vi "parseSDfeatures.vi"(0 "binary[0] string":string, 1 "binary[1] string":string) -> (9 "RESISTANCE":string, 10 "WAHOO":string, 11 "BLE":string, 12 "DEMO":string, 13 "BUZZER":string, 14 "TV":string, 15 "AUDIO":string, 16 "USB":string, 17 "FAN":string, 18 "DMK":string, 19 "DISTANCE":string, 20 "CSAFE":string, 21 "SPEED":string, 22 "byte[1] array":string[](array[string]), 23 "GRADE":string, 24 "TABLET":string, 25 "byte[0] array":string[](array[string]), 26 "PULSE":string)   [LabVIEW 2018]
uses:
  Global_1259.vi
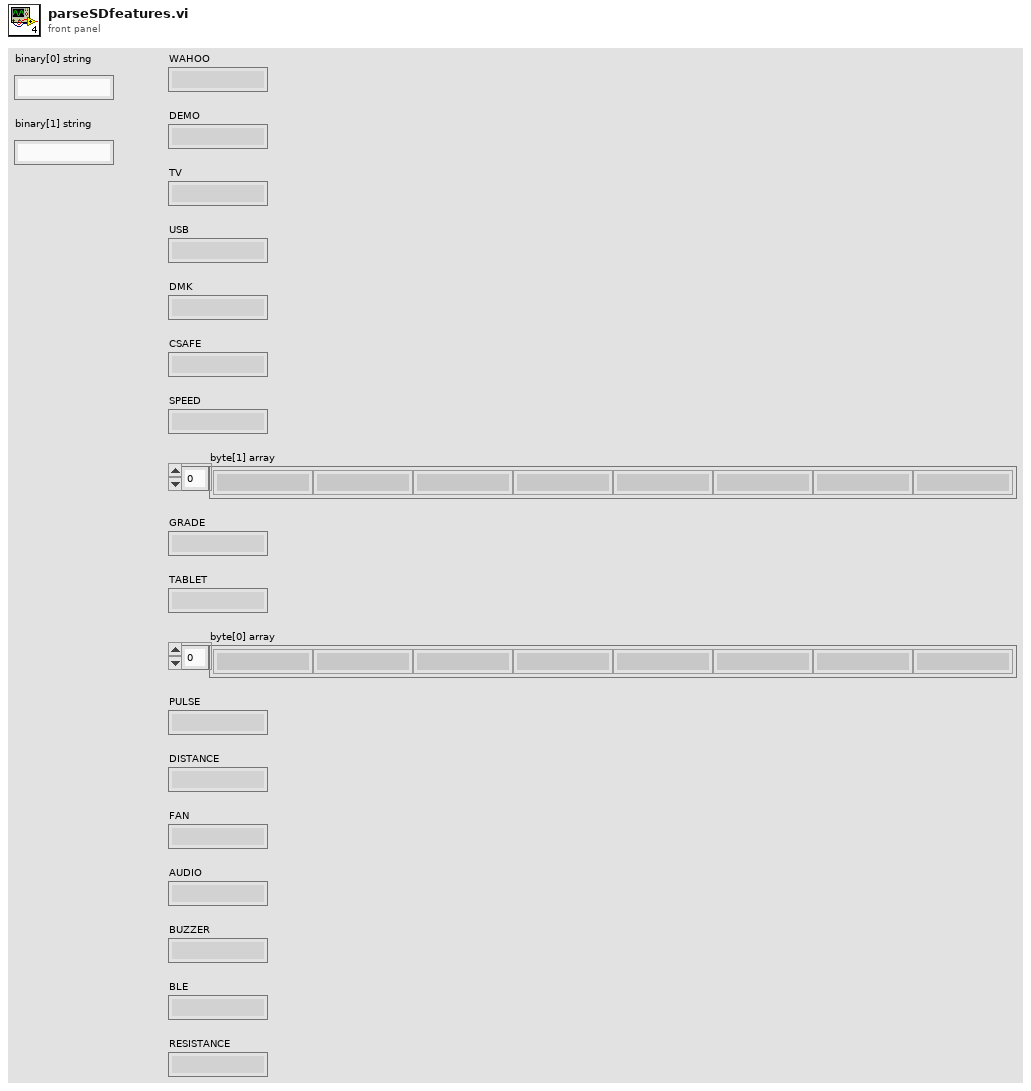
[diagram p1: front panel]
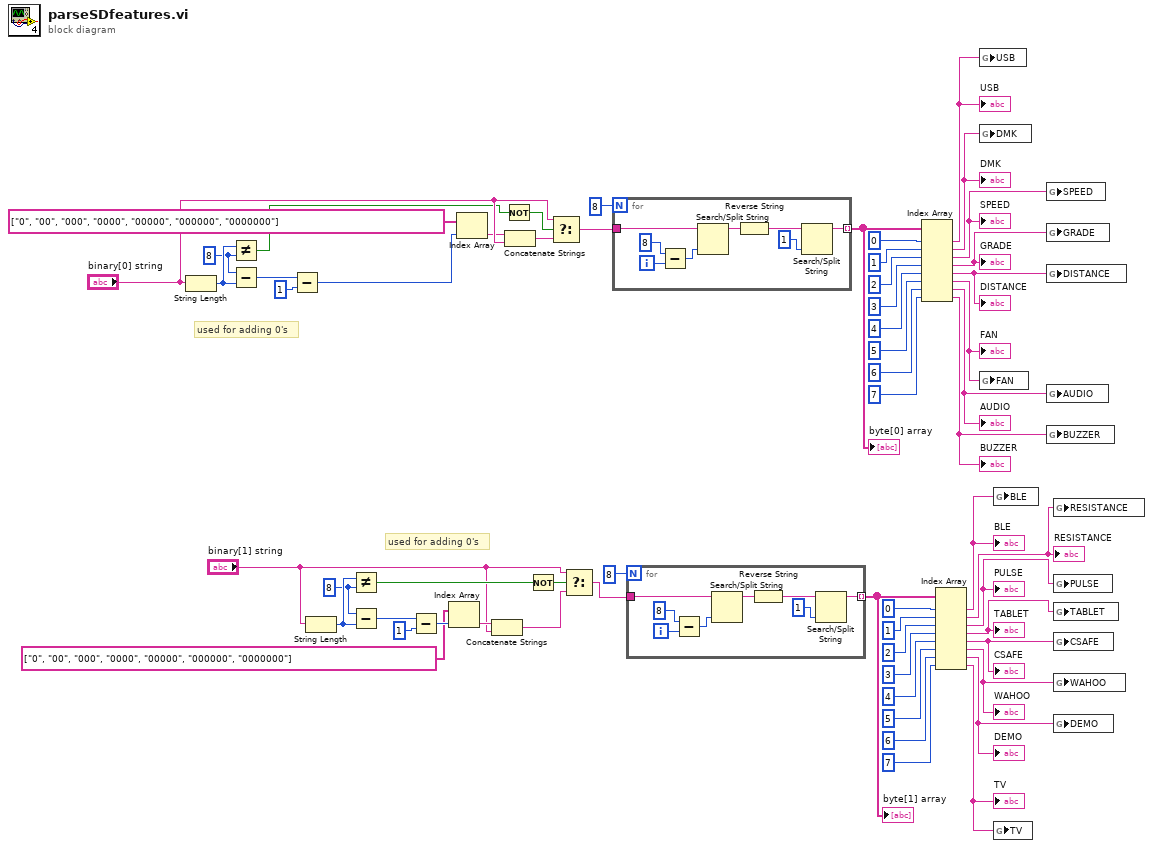
[diagram p0: block diagram]
diagram:
  w37 = 8 ("y")
  w27 = 8 ("y")
  # "used for adding 0's"
  # "used for adding 0's"
  n1 = String Length(string="binary[0] string") -> (length=w38:i32)
  n2 = Not Equal?(x=w38, y=w37) -> (x != y?=w34:bool)
  n3 = Subtract(x=w37, y=w38) -> (x-y=w40:i32)
  n4 = Subtract(x=w40, y=1) -> (x-y=w42:i32)
  n5 = String Length(string="binary[1] string") -> (length=w28:i32)
  n6 = Not Equal?(x=w28, y=w27) -> (x != y?=w24:bool)
  n7 = Subtract(x=w27, y=w28) -> (x-y=w30:i32)
  n8 = Subtract(x=w30, y=1) -> (x-y=w32:i32)
  n9 = Index Array(array=string[] ["0", "00", "000", "0000", "00000", "000000", "0000000"], index=w32) -> (element=w29:string)
  n10 = Index Array(array=string[] ["0", "00", "000", "0000", "00000", "000000", "0000000"], index=w42) -> (element=w39:string)
  n11 = Concatenate Strings(w29, "binary[1] string") -> (w22:string)
  n12 = Not(x=w34) -> (.not. x?=w35:bool)
  n13 = Concatenate Strings(w39, "binary[0] string") -> (w33:string)
  n14 = Not(x=w24) -> (.not. x?=w25:bool)
  n15 = Select(t="binary[0] string", s=w35, f=w33) -> (s? t:f=w43:string)
  n16 = Select(t="binary[1] string", s=w25, f=w22) -> (s? t:f=w21:string)
  n17 = for {
    N: 8 -> [_]
    tunnel: w43 -> [w68]
    tunnel: [w61] -> w2 mode=indexing
    i -> [w65]
    n18 = Subtract(x=8, y=w65) -> (x-y=w66:i32)
    n19 = Search/Split String(string=w68, offset (0)=w66) -> (substring before match=w64:string)  [unwired: 1 in, 2 out]
    n20 = Reverse String(1:w64) -> (0:w63:string)
    n21 = Search/Split String(string=w63, offset (0)=1) -> (substring before match=w61:string)  [unwired: 1 in, 2 out]
  }
  "byte[0] array" <- w2
  n22 = for {
    N: 8 -> [_]
    tunnel: w21 -> [w76]
    tunnel: [w69] -> w12 mode=indexing
    i -> [w73]
    n23 = Subtract(x=8, y=w73) -> (x-y=w74:i32)
    n24 = Search/Split String(string=w76, offset (0)=w74) -> (substring before match=w72:string)  [unwired: 1 in, 2 out]
    n25 = Reverse String(1:w72) -> (0:w71:string)
    n26 = Search/Split String(string=w71, offset (0)=1) -> (substring before match=w69:string)  [unwired: 1 in, 2 out]
  }
  "byte[1] array" <- w12
  n27 = Index Array(array=w2, index #1=0 ("index"), index #2=1 ("index"), index #3=2 ("index"), index #4=3 ("index"), index #5=4 ("index"), index #6=5 ("index"), index #7=6 ("index"), index #8=7 ("index")) -> (element #1=w44:string, element #2=w45:string, element #3=w46:string, element #4=w47:string, element #5=w48:string, element #6=w49:string, element #7=w50:string, element #8=w51:string)
  "SPEED" <- w46
  "GRADE" <- w47
  "DISTANCE" <- w48
  "FAN" <- w49
  "AUDIO" <- w50
  "BUZZER" <- w51
  "USB" <- w44
  "DMK" <- w45
  n28 = Index Array(array=w12, index #1=0 ("index"), index #2=1 ("index"), index #3=2 ("index"), index #4=3 ("index"), index #5=4 ("index"), index #6=5 ("index"), index #7=6 ("index"), index #8=7 ("index")) -> (element #1=w52:string, element #2=w53:string, element #3=w54:string, element #4=w55:string, element #5=w56:string, element #6=w57:string, element #7=w58:string, element #8=w59:string)
  "BLE" <- w52
  "RESISTANCE" <- w53
  "PULSE" <- w54
  "TABLET" <- w55
  "CSAFE" <- w56
  "WAHOO" <- w57
  "DEMO" <- w58
  "TV" <- w59
  n29 = global write "Global_1259.vi" "USB"(w44) -> ()
  n30 = global write "Global_1259.vi" "DMK"(w45) -> ()
  n31 = global write "Global_1259.vi" "FAN"(w49) -> ()
  n32 = global write "Global_1259.vi" "BLE"(w52) -> ()
  n33 = global write "Global_1259.vi" "TV"(w59) -> ()
  n34 = global write "Global_1259.vi" "SPEED"(w46) -> ()
  n35 = global write "Global_1259.vi" "GRADE"(w47) -> ()
  n36 = global write "Global_1259.vi" "DISTANCE"(w48) -> ()
  n37 = global write "Global_1259.vi" "AUDIO"(w50) -> ()
  n38 = global write "Global_1259.vi" "BUZZER"(w51) -> ()
  n39 = global write "Global_1259.vi" "RESISTANCE"(w53) -> ()
  n40 = global write "Global_1259.vi" "PULSE"(w54) -> ()
  n41 = global write "Global_1259.vi" "TABLET"(w55) -> ()
  n42 = global write "Global_1259.vi" "CSAFE"(w56) -> ()
  n43 = global write "Global_1259.vi" "WAHOO"(w57) -> ()
  n44 = global write "Global_1259.vi" "DEMO"(w58) -> ()
